vi "PLC控制读取.vi"(8 "error in (no error)":errorcluster caption="错误输入（无错误）", 10 "PLC指令":T2={"变量类型"=2, "PLC地址"=0, "size"=0, "写入数据(写入时有效)"=0} {"变量类型" items=["X", "Y", "M", "D"]}, 11 "PLC设置":T1) -> (0 "error out":errorcluster caption="错误输出", 1 "读取值":i16, 2 "返回值":i32, 3 "PLC设置2":T1)   [LabVIEW 2015, in "Action.lvlib"]
uses:
  Action.lvlib
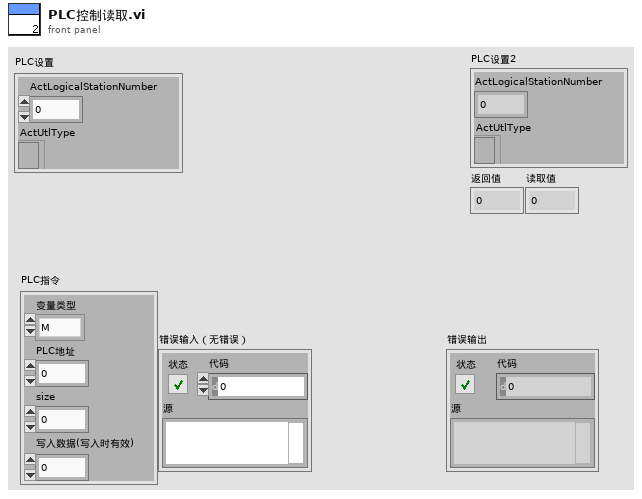
[diagram p1: front panel]
types:
  T1 = typedef "Action.lvlib/PLC设置.ctl" = cluster{"ActLogicalStationNumber":i32, "ActUtlType":refnum<k7>}
  T2 = typedef "Action.lvlib/PLC控制指令.ctl" = cluster{"变量类型":u32, "PLC地址":i32, "size":i32, "写入数据(写入时有效)":i16}
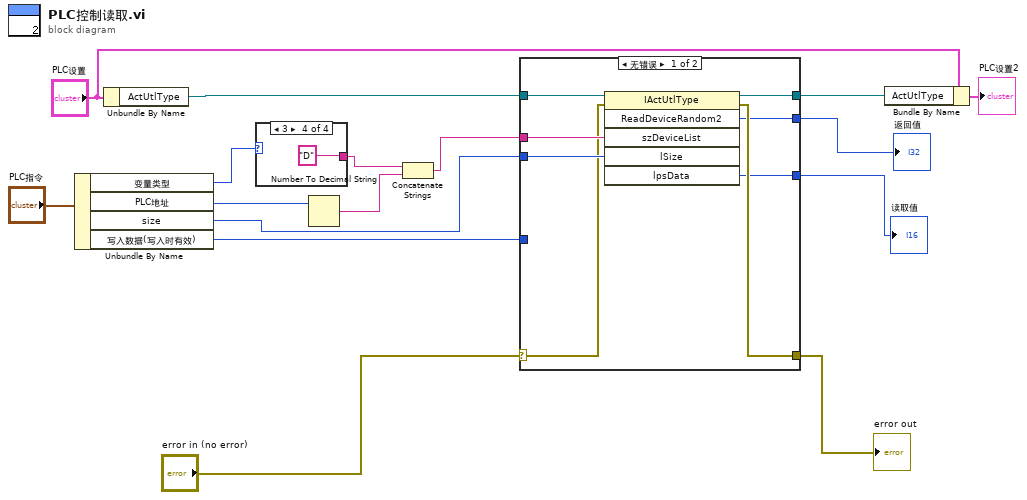
[diagram p0: block diagram]
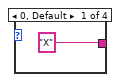
[diagram p2: hidden frame]
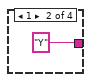
[diagram p3: hidden frame]
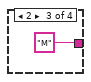
[diagram p4: hidden frame]
diagram:
  n1 = Unbundle By Name("PLC指令") -> ("变量类型"=w12:u32, "PLC地址"=w10:i32, "size"=w7:i32, "写入数据(写入时有效)"=w6:i16)
  n2 = Unbundle By Name("PLC设置") -> ("ActUtlType"=w13:refnum<k7>)
  n3 = case shown="3" w12 {
    tunnel: ["X" "Y" "M" "D"] -> w11
    frame 0, Default {
    }
    frame 1 {
    }
    frame 2 {
    }
    frame 3 {
    }
  }
  n4 = Number To Decimal String(number=w10) -> (decimal integer string=w9:string)  [unwired: 1 in]
  n5 = Concatenate Strings(w11, w9) -> (w8:string)
  n6 = case shown="无错误" "error in (no error)" {
    selector: "error in (no error)" -> [w24 w30]
    tunnel: [w23 w30] -> w14
    tunnel: w13 -> [w28 w29]
    tunnel: w8 -> [w27 _]
    tunnel: w7 -> [w26 _]
    tunnel: w6 -> [_ _]
    tunnel: [w25 w29] -> w4
    tunnel: [w22 _] -> w2
    tunnel: [w21 _] -> w1
    frame No Error {
      n7 = invoke class="IActUtlType" method="ReadDeviceRandom2"(reference=w28, error in=w24, "szDeviceList"=w27, "lSize"=w26) -> (reference out=w25:refnum<k7>, error out=w23:errorcluster, "ReadDeviceRandom2"=w22:i32, "lpsData"=w21:i16)  [unwired: 2 in, 2 out]
    }
    frame Error {
    }
  }
  "error out" <- w14
  "返回值" <- w2
  "读取值" <- w1
  n8 = Bundle By Name(cluster="PLC设置", "ActUtlType"=w4) -> (→"PLC设置2":T1)
